vi "Global percorso impostazioni.vi"() -> ()   [LabVIEW 2019]
panel:
  in  "Path settings":path=path "C:/Lavori in Corso/C2021031 VEM/Code/Settings/Impostazioni di personalizzazione"
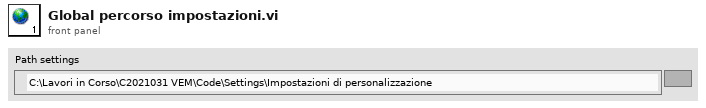
[diagram p1: front panel]
diagram:
